vi "FLImDAQ_FGV.vi"(8 "error in (no error)":errorcluster, 10 "Operation (Read)":enum16{"Write", "Read"}(ring)=enum."Read", 11 "Write data":T1={"Digitizer 1"="", "Digitizer 2"="", "Channel"=enum."Channel 0&1", "trigger source"="VAL_EXTERNAL", "trigger level"=-0.25, "trigger delay"=1.35e-07, "min sample rate"=0.5, "min record length"=0, "vertical range"=0.0, "vertical offset"=-0.25, "Waveform to Avg"=2000} {"trigger delay" format="%^#.4e"; "trigger level" min=0.0 max=3.5 step=0.5 format="%.2f"; "vertical offset" format="%.4f"; "vertical range" format="%.2f"; "min sample rate" format="%#.2p"}) -> (0 "error out":errorcluster, 3 "Read data":T1={"Digitizer 1"="", "Digitizer 2"="", "Channel"=enum."Channel 0&1", "trigger source"="VAL_EXTERNAL", "trigger level"=-0.25, "trigger delay"=1.35e-07, "min sample rate"=0.5, "min record length"=0, "vertical range"=0.0, "vertical offset"=-0.25, "Waveform to Avg"=2000} {"trigger delay" format="%^#.4e"; "trigger level" min=0.0 max=3.5 step=0.5 format="%.2f"; "vertical offset" format="%.4f"; "vertical range" format="%.2f"; "min sample rate" format="%#.2p"})   [LabVIEW 2020]
uses:
  DigitizerConfiguration/FLImDAQ.ctl
  <instrlib>/niScope/Controls/niScope trigger source.ctl
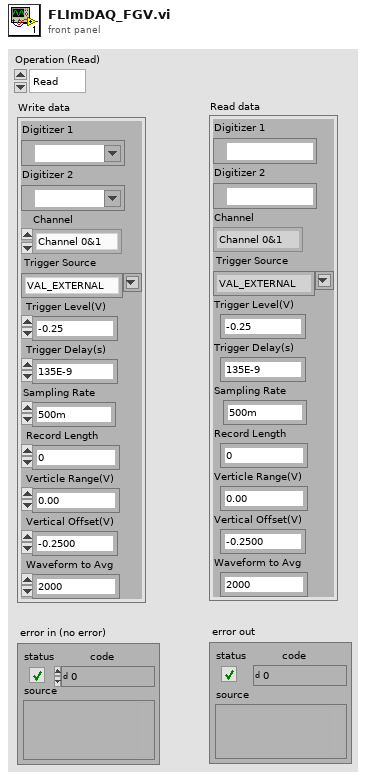
[diagram p1: front panel]
types:
  T1 = typedef "FLImDAQ.ctl" = cluster{"Digitizer 1":refnum<k15>, "Digitizer 2":refnum<k15>, "Channel":enum16{"Channel 0", "Channel 1", "Channel 0&1"}, "trigger source":T2, "trigger level":dbl, "trigger delay":dbl, "min sample rate":dbl, "min record length":i32, "vertical range":dbl, "vertical offset":dbl, "Waveform to Avg":i16}
  T2 = typedef "niScope trigger source.ctl" = string
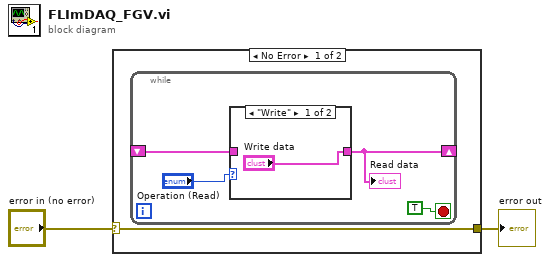
[diagram p0: block diagram]
diagram:
  n1 = case shown="No Error" "error in (no error)" {
    selector: "error in (no error)" -> [w3 w10]
    tunnel: [w3 w10] -> w1
    frame No Error {
      n2 = while {
        shift-right: [w5] -> _
        shift-left: _ -> [w4]
        stop <- TRUE stop-if-true
        n3 = case shown="\"Write\"" "Operation (Read)" {
          tunnel: ["Write data" w9] -> w5
          tunnel: w4 -> [_ w9]
          frame "Write" {
          }
          frame "Read", Default {
          }
        }
        "Read data" <- w5
      }
    }
    frame Error {
    }
  }
  "error out" <- w1
